vi "_Create Data Queeue.vi"(7 "max queue size (-1, unlimited)":i32=-1, 8 "error in (no error)":errorcluster, 9 "create if not found? (T)":bool=TRUE, 11 "Name":string) -> (0 "error out":errorcluster, 1 "created new?":bool, 3 "Queue out":refnum<queue>)   [LabVIEW 2020]
uses:
  Def-Cross JKI StateMachine State Data.ctl
  Def-Cross JKI StateMachine State Response.ctl
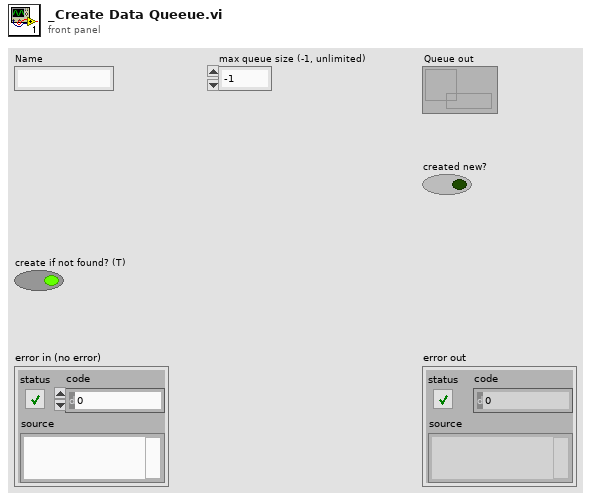
[diagram p1: front panel]
types:
  T1 = typedef "Def-Cross JKI StateMachine State Data.ctl" = cluster{"state":string, "args":string, "source":string, "RespQ":refnum<queue>}
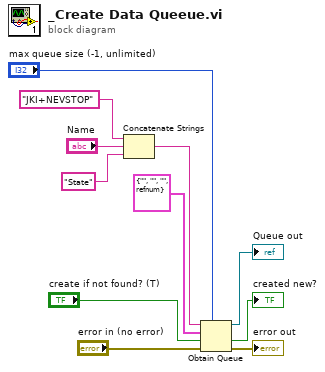
[diagram p0: block diagram]
diagram:
  n1 = Concatenate Strings("JKI+NEVSTOP" ("string"), "Name", "State" ("string in")) -> (w8:string)
  n2 = Obtain Queue(max queue size (-1, unlimited)="max queue size (-1, unlimited)", name (unnamed)=w8, element data type=T1 {"state"="", "args"="", "source"="", "RespQ"=refnum} ("Cross JKI State Machine State"), create if not found? (T)="create if not found? (T)", error in (no error)="error in (no error)") -> (queue out=→"Queue out":refnum<queue>, created new?=→"created new?":bool, error out=→"error out":errorcluster)
